vi "LED_Perform Measurements.vi"(8 "error in":errorcluster, 9 "Voltage Values":dbl[](array[numeric]), 11 "Measurement Config_In":T1={"Load channel name"="", "Load out"="", "Source out"="", "Source channel name"="", "Source sequence name"="", "Voltage values"=[], "Voltage values-CV"=[], "Voltage values-LED"=[], "Output Resistance-LED"=[], "Source terminal name"="", "Measure terminal name"="", "Load Voltage-out"=[], "Load Current - out"=[], "Source Voltage-out"=[], "Source Current - out"=[], "LED Mode Start?"=FALSE, "LED Mode Completed?"=FALSE, "CalculateRd"=0.0, "Set LED Current Limit?"=FALSE, "OutputVoltageOffset"=0.0, "measurement results"={"Status"="Empty", "Source voltages"=[0.0], "Load voltages"=[0.0], "Source Current"=[0.0], "Load Current"=[0.0]}}) -> (0 "error Out":errorcluster, 1 "Measurement Data":T3, 3 "Measurement Config_Out":T1={"Load channel name"="", "Load out"="", "Source out"="", "Source channel name"="", "Source sequence name"="", "Voltage values"=[], "Voltage values-CV"=[], "Voltage values-LED"=[], "Output Resistance-LED"=[], "Source terminal name"="", "Measure terminal name"="", "Load Voltage-out"=[], "Load Current - out"=[], "Source Voltage-out"=[], "Source Current - out"=[], "LED Mode Start?"=FALSE, "LED Mode Completed?"=FALSE, "CalculateRd"=0.0, "Set LED Current Limit?"=FALSE, "OutputVoltageOffset"=0.0, "measurement results"={"Status"="Empty", "Source voltages"=[0.0], "Load voltages"=[0.0], "Source Current"=[0.0], "Load Current"=[0.0]}})   [LabVIEW 2021, in "Startup.lvlib"]
doc: "This VI captures the Measurement data from Source and Load, for the Input Voltage."
uses:
  Startup.lvlib
  Controls/LEDStartup_Data.ctl
  Measurement Results.ctl
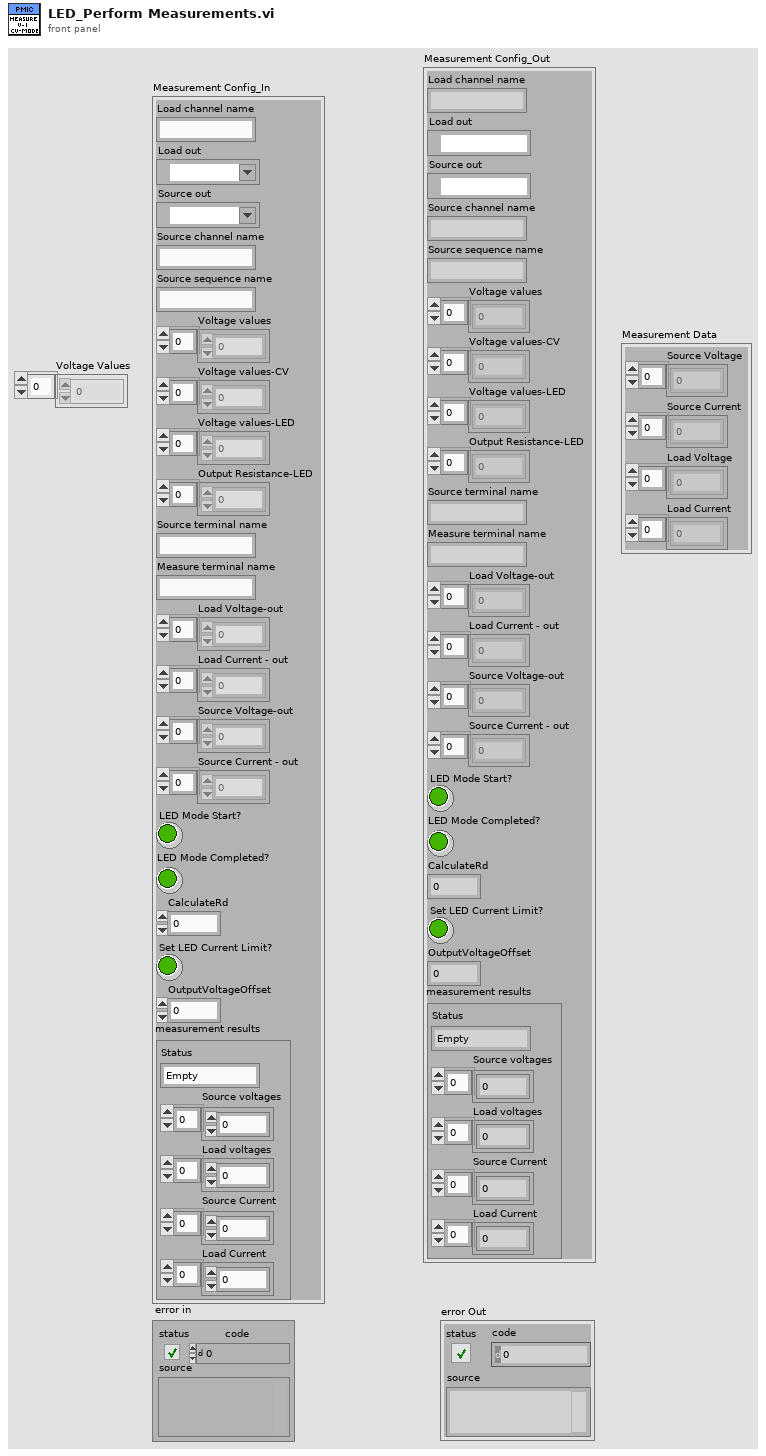
[diagram p1: front panel]
types:
  T1 = typedef "Startup.lvlib/LEDStartup_Data.ctl" = cluster{"Load channel name":string, "Load out":refnum<k15>, "Source out":refnum<k15>, "Source channel name":string, "Source sequence name":string, "Voltage values":dbl[], "Voltage values-CV":dbl[], "Voltage values-LED":dbl[], "Output Resistance-LED":dbl[], "Source terminal name":string, "Measure terminal name":string, "Load Voltage-out":dbl[], "Load Current - out":dbl[], "Source Voltage-out":dbl[], "Source Current - out":dbl[], "LED Mode Start?":bool, "LED Mode Completed?":bool, "CalculateRd":dbl, "Set LED Current Limit?":bool, "OutputVoltageOffset":dbl, "measurement results":T2}
  T2 = typedef "Startup.lvlib/Measurement Results.ctl" = cluster{"Status":string, "Source voltages":dbl[], "Load voltages":dbl[], "Source Current":dbl[], "Load Current":dbl[]}
  T3 = cluster{"Source Voltage":dbl[], "Source Current":dbl[], "Load Voltage":dbl[], "Load Current":dbl[]}
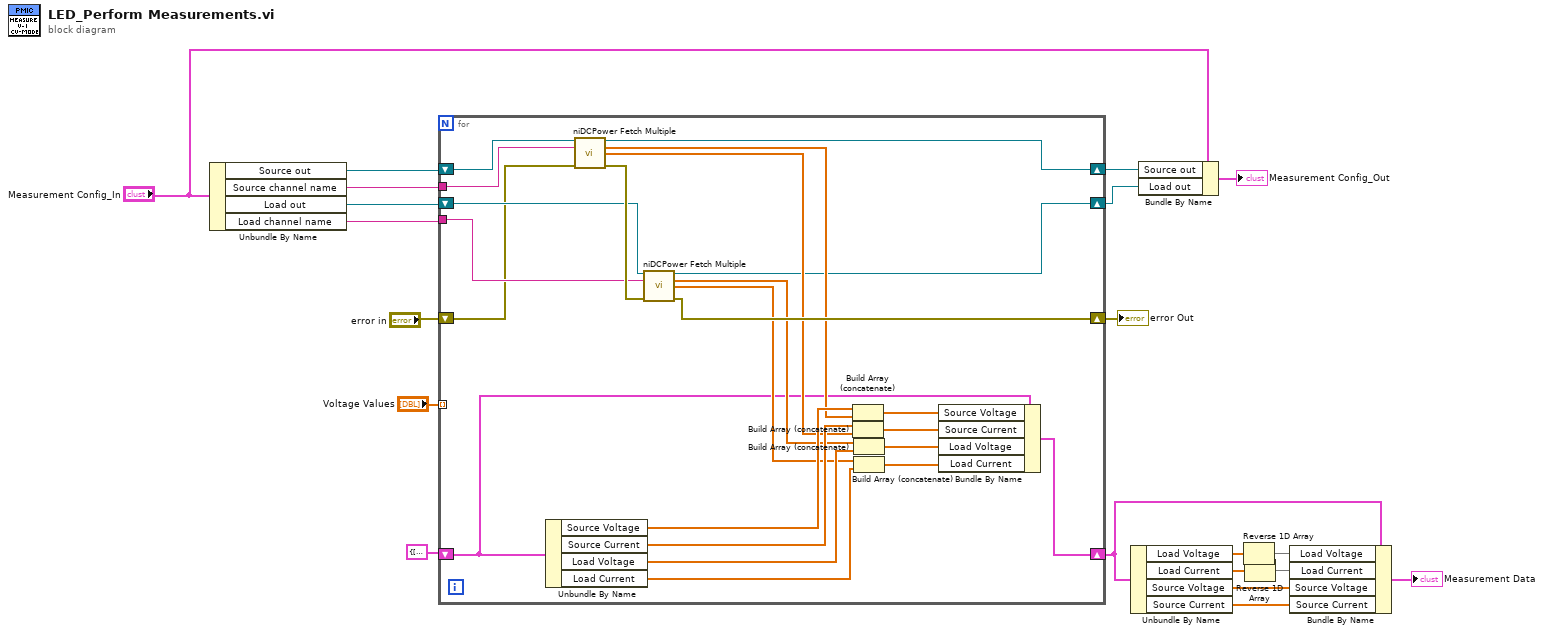
[diagram p0: block diagram]
diagram:
  n1 = Unbundle By Name("Measurement Config_In") -> ("Source out"=w20:refnum<k15>, "Source channel name"=w18:string, "Load out"=w19:refnum<k15>, "Load channel name"=w17:string)
  n2 = for {
    tunnel: w18 -> [w41]
    tunnel: w17 -> [w40]
    shift-right: [w39] -> w16
    shift-left: "error in" -> [w23]
    shift-right: [w24] -> w11
    shift-left: T3 {"Source Voltage"=[], "Source Current"=[], "Load Voltage"=[], "Load Current"=[]} -> [w29]
    tunnel: "Voltage Values" -> [_] mode=indexing
    shift-right: [w22] -> w7
    shift-left: w20 -> [w42]
    shift-right: [w21] -> w6
    shift-left: w19 -> [w38]
    n3 = Unbundle By Name(w29) -> ("Source Voltage"=w37:dbl[], "Source Current"=w35:dbl[], "Load Voltage"=w32:dbl[], "Load Current"=w30:dbl[])
    n4 = call <instrlib>:"niDCPower Fetch Multiple.vi"("instrument handle"=w42, "channel name"=w41, "error in (no error)"=w23) -> ("instrument handle out"=w22:refnum<k15>, "voltage measurements"=w36:dbl[], "current measurements"=w34:dbl[], "error out"=w43:errorcluster)  [unwired: 2 in, 7 out]
    n5 = call <instrlib>:"niDCPower Fetch Multiple.vi"("instrument handle"=w38, "channel name"=w40, "error in (no error)"=w43) -> ("instrument handle out"=w21:refnum<k15>, "voltage measurements"=w33:dbl[], "current measurements"=w31:dbl[], "error out"=w39:errorcluster)  [unwired: 2 in, 7 out]
    n6 = Build Array (concatenate)(w37, w36) -> (w28:dbl[])
    n7 = Build Array (concatenate)(w35, w34) -> (w27:dbl[])
    n8 = Build Array (concatenate)(w33, w32) -> (w26:dbl[])
    n9 = Build Array (concatenate)(w31, w30) -> (w25:dbl[])
    n10 = Bundle By Name(cluster=w29, "Source Voltage"=w28, "Source Current"=w27, "Load Voltage"=w26, "Load Current"=w25) -> (w24:T3)
  }
  "error Out" <- w16
  n11 = Unbundle By Name(w11) -> ("Load Voltage"=w13:dbl[], "Load Current"=w12:dbl[], "Source Voltage"=w5:dbl[], "Source Current"=w4:dbl[])
  n12 = Bundle By Name(cluster="Measurement Config_In", "Source out"=w7, "Load out"=w6) -> (→"Measurement Config_Out":T1)
  n13 = Reverse 1D Array(array=w13) -> (reversed array=w10:dbl[])
  n14 = Reverse 1D Array(array=w12) -> (reversed array=w9:dbl[])
  n15 = Bundle By Name(cluster=w11, "Load Voltage"=w10, "Load Current"=w9, "Source Voltage"=w5, "Source Current"=w4) -> (→"Measurement Data":T3)
